vi "TransformToDiff.vi"   [LabVIEW 2017, in "NI_Kinematics.lvlib"]
uses:
  <vilib>/robotics/Kinematics/NI_Kinematics.lvlib
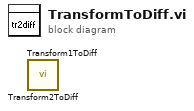
[diagram p0: block diagram]
diagram:
  n1 = call <vilib>:"Transform2ToDiff.vi"() -> ()  [unwired: 2 in, 1 out]
  n2 = call <vilib>:"Transform1ToDiff.vi"() -> ()  [unwired: 2 in, 1 out]
